vi "Main Report.vi"() -> ()   [LabVIEW 2014]
uses:
  <vilib>/addons/database/Connection.llb/DB Tools Open Connec (String).vi
  <vilib>/Utility/NIReport.llb/Append Text Table to Report (wrap).vi
  <vilib>/Utility/NIReport.llb/Append Numeric Table to Report (wrap).vi
  <vilib>/Utility/NIReport.llb/NI_report.lvclass
  <vilib>/addons/database/NI_Database_API.lvlib
  FIRST Reports.lvlib
  <vilib>/Utility/NIReport.llb/Excel/NI_Excel.lvclass
  <vilib>/National Instruments/LabVIEW Interface for Amazon S3/Typedefs/AMZ_S3_AWS Credentials.ctl
panel:
  out "error out":errorcluster
  in  "error in (no error)":errorcluster
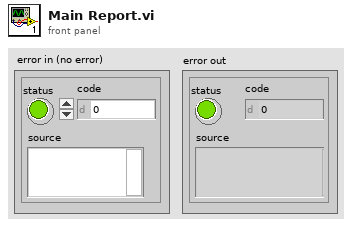
[diagram p1: front panel]
types:
  T1 = cluster{"left":i32, "top":i32, "height":dbl, "width":dbl}
  T2 = cluster{"position (excel)":cluster{"row":i32, "column":i32}, "name (excel)":string, "bookmark (word)":string}
  T3 = enum16{"Standard Report", "HTML", "Word", "Excel"}
  T4 = typedef "NI_Database_API.lvlib/Conn ObjectReference.ctl" = refnum<k1>
  T5 = typedef "LV Interface for Amazon S3.lvlib/AMZ_S3_AWS Credentials.ctl" = cluster{"Access Key":string, "Secret Key":string}
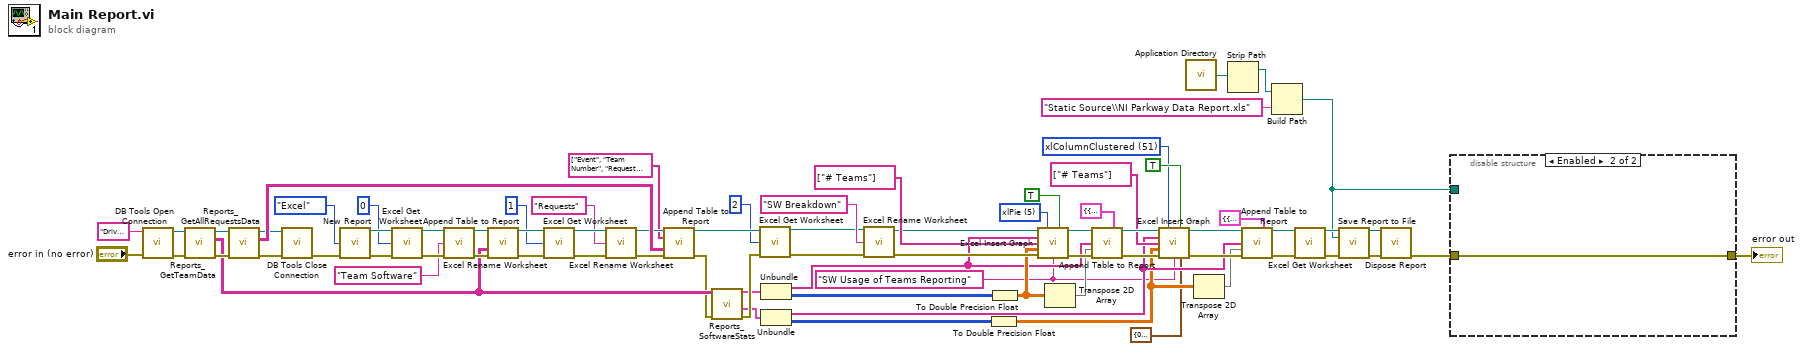
[diagram p0: block diagram]
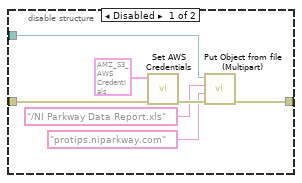
[diagram p2: hidden frame]
diagram:
  w22 = 51 items=["xlColumnClustered"=51, "xlColumnStacked"=52, "xlColumnStacked100"=53, "xl3DColumnClustered"=54, "xl3DColumnStacked"=55, "xl3DColumnStacked100"=56, "xlBarClustered"=57, "xlBarStacked"=58, "xlBarStacked100"=59, "xl3DBarClustered"=60, "xl3DBarStacked"=61, "xl3DBarStacked100"=62, "xlLineStacked"=63, "xlLineStacked100"=64, "xlLineMarkers"=65, "xlLineMarkersStacked"=66, "xlLineMarkersStacked100"=67, "xlPieOfPie"=68, "xlPieExploded"=69, "xl3DPieExploded"=70, "xlBarOfPie"=71, "xlXYScatterSmooth"=72, "xlXYScatterSmoothNoMarkers"=73, "xlXYScatterLines"=74, "xlXYScatterLinesNoMarkers"=75, "xlAreaStacked"=76, "xlAreaStacked100"=77, "xl3DAreaStacked"=78, "xl3DAreaStacked100"=79, "xlDoughnutExploded"=80, "xlRadarMarkers"=81, "xlRadarFilled"=82, "xlSurface"=83, "xlSurfaceWireframe"=84, "xlSurfaceTopView"=85, "xlSurfaceTopViewWireframe"=86, "xlBubble"=15, "xlBubble3DEffect"=87, "xlStockHLC"=88, "xlStockOHLC"=89, "xlStockVHLC"=90, "xlStockVOHLC"=91, "xlCylinderColClustered"=92, "xlCylinderColStacked"=93, "xlCylinderColStacked100"=94, "xlCylinderBarClustered"=95, "xlCylinderBarStacked"=96, "xlCylinderBarStacked100"=97, "xlCylinderCol"=98, "xlConeColClustered"=99, "xlConeColStacked"=100, "xlConeColStacked100"=101, "xlConeBarClustered"=102, "xlConeBarStacked"=103, "xlConeBarStacked100"=104, "xlConeCol"=105, "xlPyramidColClustered"=106, "xlPyramidColStacked"=107, "xlPyramidColStacked100"=108, "xlPyramidBarClustered"=109, "xlPyramidBarStacked"=110, "xlPyramidBarStacked100"=111, "xlPyramidCol"=112, "xl3DColumn"=-4100, "xlLine"=4, "xl3DLine"=-4101, "xl3DPie"=-4102, "xlPie"=5, "xlXYScatter"=-4169, "xl3DArea"=-4098, "xlArea"=1, "xlDoughnut"=-4120, "xlRadar"=-4151] ("graph type (col clustered)")
  w12 = "SW Usage of Teams Reporting" ("graph title (\"\")")
  w40 = 5 items=["xlColumnClustered"=51, "xlColumnStacked"=52, "xlColumnStacked100"=53, "xl3DColumnClustered"=54, "xl3DColumnStacked"=55, "xl3DColumnStacked100"=56, "xlBarClustered"=57, "xlBarStacked"=58, "xlBarStacked100"=59, "xl3DBarClustered"=60, "xl3DBarStacked"=61, "xl3DBarStacked100"=62, "xlLineStacked"=63, "xlLineStacked100"=64, "xlLineMarkers"=65, "xlLineMarkersStacked"=66, "xlLineMarkersStacked100"=67, "xlPieOfPie"=68, "xlPieExploded"=69, "xl3DPieExploded"=70, "xlBarOfPie"=71, "xlXYScatterSmooth"=72, "xlXYScatterSmoothNoMarkers"=73, "xlXYScatterLines"=74, "xlXYScatterLinesNoMarkers"=75, "xlAreaStacked"=76, "xlAreaStacked100"=77, "xl3DAreaStacked"=78, "xl3DAreaStacked100"=79, "xlDoughnutExploded"=80, "xlRadarMarkers"=81, "xlRadarFilled"=82, "xlSurface"=83, "xlSurfaceWireframe"=84, "xlSurfaceTopView"=85, "xlSurfaceTopViewWireframe"=86, "xlBubble"=15, "xlBubble3DEffect"=87, "xlStockHLC"=88, "xlStockOHLC"=89, "xlStockVHLC"=90, "xlStockVOHLC"=91, "xlCylinderColClustered"=92, "xlCylinderColStacked"=93, "xlCylinderColStacked100"=94, "xlCylinderBarClustered"=95, "xlCylinderBarStacked"=96, "xlCylinderBarStacked100"=97, "xlCylinderCol"=98, "xlConeColClustered"=99, "xlConeColStacked"=100, "xlConeColStacked100"=101, "xlConeBarClustered"=102, "xlConeBarStacked"=103, "xlConeBarStacked100"=104, "xlConeCol"=105, "xlPyramidColClustered"=106, "xlPyramidColStacked"=107, "xlPyramidColStacked100"=108, "xlPyramidBarClustered"=109, "xlPyramidBarStacked"=110, "xlPyramidBarStacked100"=111, "xlPyramidCol"=112, "xl3DColumn"=-4100, "xlLine"=4, "xl3DLine"=-4101, "xl3DPie"=-4102, "xlPie"=5, "xlXYScatter"=-4169, "xl3DArea"=-4098, "xlArea"=1, "xlDoughnut"=-4120, "xlRadar"=-4151] ("graph type (col clustered)")
  n1 = call-poly <vilib>:"DB Tools Open Connection.vi"("error in (no error)"="error in (no error)", "connection information"="Driver={MySQL ODBC 5.2w Driver};Server=parkway-production.cjlclmebggwl.us-east-1.rds.amazonaws.com;Database=parkway;User=parkway;Password=moonlightmarj;" ("Connection String")) -> ("error out"=w47:errorcluster, "connection reference"=w52:T4)  [unwired: 6 in]
  n2 = call "Reports_GetTeamData.vi"("error in (no error)"=w47, "Refnum in"=w52) -> ("error out"=w51:errorcluster, "Array"=w46:string[][], "Refnum Out"=w50:T4)  [unwired: 7 in]
  n3 = call "Reports_GetAllRequestsData.vi"("error in (no error)"=w51, "Refnum in"=w50) -> ("error out"=w48:errorcluster, "Array"=w76:string[][], "Refnum Out"=w49:T4)  [unwired: 7 in]
  n4 = call <vilib>:"DB Tools Close Connection.vi"("error in (no error)"=w48, "connection reference"=w49) -> ("error out"=w75:errorcluster)  [unwired: 5 in]
  n5 = call <vilib>:"New Report.vi"("report type"=T3."Excel", "error in (no error)"=w75) -> ("report out"=w73:refnum<class "NI_report.lvclass">, "error out"=w72:errorcluster)  [unwired: 12 in]
  n6 = call <vilib>:"Excel Get Worksheet.vi"("report in"=w73, "worksheet index (0)"=0, "error in (no error)"=w72) -> ("report out"=w70:refnum<class "NI_report.lvclass">, "error out"=w69:errorcluster)  [unwired: 11 in]
  n7 = call <vilib>:"Excel Rename Worksheet.vi"("report in"=w70, "worksheet name (\"\")"="Team Software" ("worksheet name (\"\")"), "error in (no error)"=w69) -> ("report out"=w65:refnum<class "NI_report.lvclass">, "error out"=w64:errorcluster)  [unwired: 11 in]
  n8 = call-poly <vilib>:"Append Table to Report.vi"("report in"=w65, "text data"=w46, "error in (no error)"=w64) -> ("report out"=w60:refnum<class "NI_report.lvclass">, "error out"=w63:errorcluster)  [unwired: 9 in, 2 out]
  n9 = call <vilib>:"Excel Get Worksheet.vi"("report in"=w60, "worksheet index (0)"=1, "error in (no error)"=w63) -> ("report out"=w59:refnum<class "NI_report.lvclass">, "error out"=w62:errorcluster)  [unwired: 11 in]
  n10 = call <vilib>:"Excel Rename Worksheet.vi"("report in"=w59, "worksheet name (\"\")"="Requests" ("worksheet name (\"\")"), "error in (no error)"=w62) -> ("report out"=w58:refnum<class "NI_report.lvclass">, "error out"=w61:errorcluster)  [unwired: 11 in]
  n11 = call-poly <vilib>:"Append Table to Report.vi"("report in"=w58, "column headers"=string[] ["Event", "Team Number", "Request Number", "Request Status", "Request Text ", "Open Date", "Close Date", "Solution Text", "Request URL"], "text data"=w76, "error in (no error)"=w61) -> ("report out"=w54:refnum<class "NI_report.lvclass">, "error out"=w33:errorcluster)  [unwired: 8 in, 2 out]
  n12 = call "Reports_SoftwareStats.vi"("Error In"=w33, "All Team Software Data"=w46) -> ("Error Out"=w32:errorcluster, "Add-On SW Stats"=w26:cluster{"Add-On Types":string[], i32[][]}, "Main SW Stats"=w29:cluster{string[], i32[][]})  [unwired: 7 in]
  n13 = call <vilib>:"Excel Get Worksheet.vi"("report in"=w54, "worksheet index (0)"=2, "error in (no error)"=w32) -> ("report out"=w42:refnum<class "NI_report.lvclass">, "error out"=w41:errorcluster)  [unwired: 11 in]
  n14 = Unbundle(w29) -> (w28:string[], w27:i32[][])
  n15 = Unbundle(w26) -> ("Add-On Types"=w17:string[], w20:i32[][])
  n16 = call <vilib>:"Excel Rename Worksheet.vi"("report in"=w42, "worksheet name (\"\")"="SW Breakdown" ("worksheet name (\"\")"), "error in (no error)"=w41) -> ("report out"=w39:refnum<class "NI_report.lvclass">, "error out"=w38:errorcluster)  [unwired: 11 in]
  n17 = To Double Precision Float(number=w20) -> (double precision float=w16:dbl[][])
  n18 = To Double Precision Float(number=w27) -> (double precision float=w31:dbl[][])
  n19 = call <vilib>:"Excel Insert Graph.vi"("report in"=w39, "graph type (col clustered)"=w40, "has legend? (F)"=TRUE, "column headers"=w28, "row headers"=string[] ["# Teams"], "data"=w31, "error in (no error)"=w38, "graph title (\"\")"=w12) -> ("report out"=w36:refnum<class "NI_report.lvclass">, "error out"=w35:errorcluster)  [unwired: 6 in]
  n20 = Transpose 2D Array(2D array=w31) -> (transposed array=w30:dbl[][])
  n21 = call-poly <vilib>:"Append Table to Report.vi"("report in"=w36, "MS Office parameters"=T2 {"position (excel)"={"row"=20, "column"=0}, "name (excel)"="", "bookmark (word)"=""}, "row headers"=w28, "numerical data"=w30, "error in (no error)"=w35) -> ("report out"=w25:refnum<class "NI_report.lvclass">, "error out"=w24:errorcluster)  [unwired: 7 in, 2 out]
  n22 = call <vilib>:"Excel Insert Graph.vi"("report in"=w25, "graph type (col clustered)"=w22, "has legend? (F)"=TRUE, "column headers"=w17, "row headers"=string[] ["# Teams"], "data"=w16, "error in (no error)"=w24, "graph title (\"\")"=w12, "position/size"=T1 {"left"=0, "top"=6, "height"=4.0, "width"=4.0}) -> ("report out"=w19:refnum<class "NI_report.lvclass">, "error out"=w18:errorcluster)  [unwired: 5 in]
  n23 = call <vilib>:"Application Directory.vi"() -> ("Application Directory"=w3:path)
  n24 = Transpose 2D Array(2D array=w16) -> (transposed array=w15:dbl[][])
  n25 = Strip Path(path=w3) -> (stripped path=w2:path)  [unwired: 1 out]
  n26 = call-poly <vilib>:"Append Table to Report.vi"("report in"=w19, "MS Office parameters"=T2 {"position (excel)"={"row"=20, "column"=6}, "name (excel)"="", "bookmark (word)"=""}, "row headers"=w17, "numerical data"=w15, "error in (no error)"=w18) -> ("report out"=w9:refnum<class "NI_report.lvclass">, "error out"=w8:errorcluster)  [unwired: 7 in, 2 out]
  n27 = Build Path(base path=w2, name or relative path="Static Source\\NI Parkway Data Report.xls") -> (appended path=w1:path)
  n28 = call <vilib>:"Excel Get Worksheet.vi"("report in"=w9, "error in (no error)"=w8) -> ("report out"=w11:refnum<class "NI_report.lvclass">, "error out"=w10:errorcluster)  [unwired: 12 in]
  n29 = call-dynamic "Save Report to File.vi"("report in"=w11, "report file path"=w1, "error in (no error)"=w10) -> ("report out"=w67:refnum<class "NI_report.lvclass">, "error out"=w66:errorcluster)  [unwired: 11 in]
  n30 = call-dynamic "Dispose Report.vi"("report in"=w67, "error in (no error)"=w66) -> ("error out"=w7:errorcluster)  [unwired: 13 in]
  n31 = disable-structure shown="Enabled" {
    disable-tunnel: w7 -> [w81 w84]
    disable-tunnel: w1 -> [w80 _]
    disable-tunnel: [w77 w84] -> w4
    frame Disabled {
      n32 = call <vilib>:"Set AWS Credentials.vi"("error in (no error)"=w81, "AWS Credentials in"=T5 {"Access Key"="AKIAI4UOFGXQQ2XM3KTQ", "Secret Key"="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"}) -> ("error out"=w82:errorcluster)  [unwired: 9 in]
      n33 = call <vilib>:"Put Object from file (Multipart).vi"("error in (no error)"=w82, "Bucket"="protips.niparkway.com", "Object path"="/NI Parkway Data Report.xls", "Local file path"=w80) -> ("error out"=w77:errorcluster)  [unwired: 5 in, 2 out]
    }
    frame Enabled {
    }
  }
  "error out" <- w4
